vi "状态告警区.vi"(11 "数组":u16[](array[numeric]) format="%04xH") -> (2 "状态告警区 2":T1 {"工作状态" items=["空闲"=0, "水样测试"=1, "标样核查"=2, "零点核查"=3, "跨度核查"=4, "空白测试"=5, "平行样测试"=6, "加标回收"=7, "空白校准"=8, "标样校准"=9, "初始化（清洗）"=10, "单步调试"=254, "简易步骤"=255]; "告警代码" items=["无告警", "缺试剂告警", "缺水样告警", "缺蒸馏水告警", "缺标液告警", "仪表漏液告警", "标定异常告警", "超量程告警", "加热异常", "低试剂预警", "超上限告警", "超下限告警", "仪表内部其他异常", "滴定异常告警", "电极异常告警", "量程切换告警", "参数设置告警", "PH电极电位异常", "电导率电极异常", "浊度光度异常", "溶解氧电极异常", "溶解氧光强异常", "温度异常告警", "PH异常告警", "溶解氧异常告警", "电导率异常告警", "浊度异常告警", "叶绿素异常告警", "藻密度异常告警", "蓝绿藻异常告警", "ORP异常告警", "氨氮异常告警", "清洁刷异常告警", "SD卡异常告警", "蓝牙异常告警", "Wifi异常告警", "流程异常告警"]; "故障代码" items=["无故障", "电机故障", "温度故障", "通讯故障", "滴定故障"]}, 3 "状态告警区":T2 {"工作状态" items=["空闲"=0, "水样测试"=1, "标样核查"=2, "零点核查"=3, "跨度核查"=4, "空白测试"=5, "平行样测试"=6, "加标回收"=7, "空白校准"=8, "标样校准"=9, "初始化（清洗）"=10, "单步调试"=254, "简易步骤"=255]; "告警代码" items=["无告警", "缺试剂告警", "缺水样告警", "缺蒸馏水告警", "缺标液告警", "仪表漏液告警", "标定异常告警", "超量程告警", "加热异常", "低试剂预警", "超上限告警", "超下限告警", "仪表内部其他异常", "滴定异常告警", "电极异常告警", "量程切换告警", "参数设置告警", "PH电极电位异常", "电导率电极异常", "浊度光度异常", "溶解氧电极异常", "溶解氧光强异常", "温度异常告警", "PH异常告警", "溶解氧异常告警", "电导率异常告警", "浊度异常告警", "叶绿素异常告警", "藻密度异常告警", "蓝绿藻异常告警", "ORP异常告警", "氨氮异常告警", "清洁刷异常告警", "SD卡异常告警", "蓝牙异常告警", "Wifi异常告警", "流程异常告警"]; "故障代码" items=["无故障", "电机故障", "温度故障", "通讯故障", "滴定故障"]})   [LabVIEW 2022 SP3, in "斯坦道通用流路CODmn.lvlib"]
panel:
  # "共占用29 WORD"
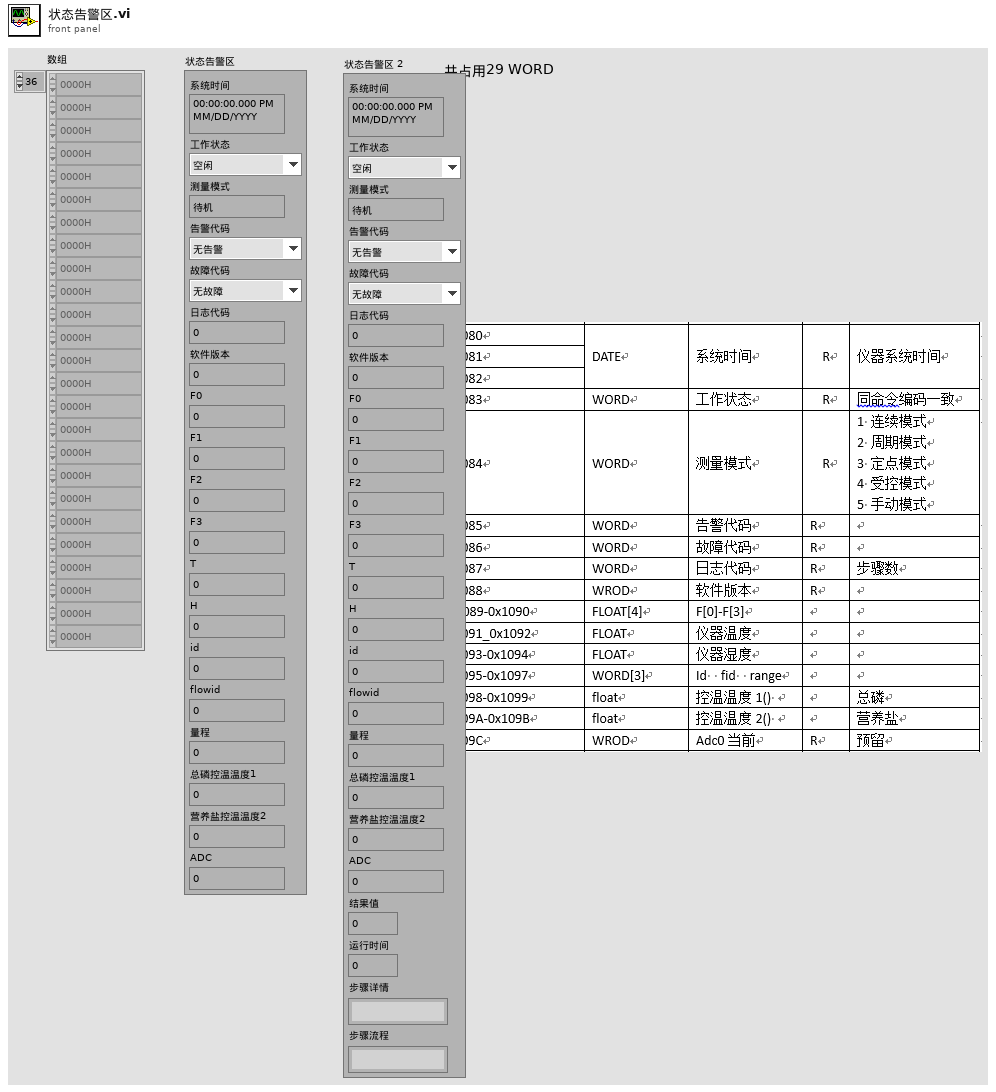
[diagram p1: front panel]
types:
  T1 = cluster{"系统时间":timestamp, "工作状态":u16, "测量模式":enum16{"待机", "连续模式", "周期模式", "定点模式", "受控模式", "手动模式"}, "告警代码":u16, "故障代码":u16, "日志代码":u16, "软件版本":u16, "F0":sgl, "F1":sgl, "F2":sgl, "F3":sgl, "T":sgl, "H":sgl, "id":u16, "flowid":u16, "量程":u16, "总磷控温温度1":sgl, "营养盐控温温度2":sgl, "ADC":sgl, "结果值":sgl, "运行时间":u16, "步骤详情":string, "步骤流程":string}
  T2 = cluster{"系统时间":timestamp, "工作状态":u16, "测量模式":enum16{"待机", "连续模式", "周期模式", "定点模式", "受控模式", "手动模式"}, "告警代码":u16, "故障代码":u16, "日志代码":u16, "软件版本":u16, "F0":sgl, "F1":sgl, "F2":sgl, "F3":sgl, "T":sgl, "H":sgl, "id":u16, "flowid":u16, "量程":u16, "总磷控温温度1":sgl, "营养盐控温温度2":sgl, "ADC":sgl}
  T3 = enum16{"待机", "连续模式", "周期模式", "定点模式", "受控模式", "手动模式"}
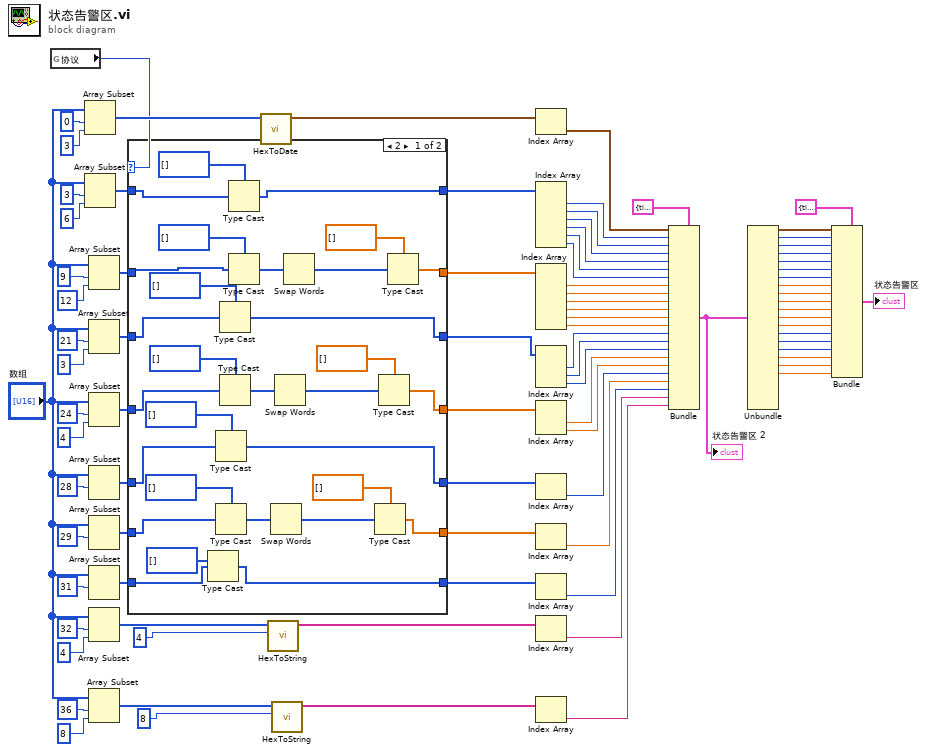
[diagram p0: block diagram]
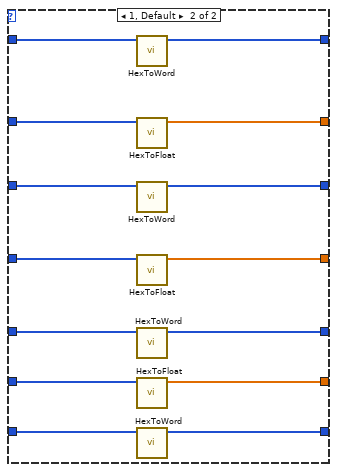
[diagram p2: hidden frame]
diagram:
  n1 = global read "总磷总氮断电保存全局变量.vi" "协议"() -> (w1:u16)
  n2 = Array Subset(array="数组", index=0 ("索引"), length=3 ("长度")) -> (w85:u16[])
  n3 = Array Subset(array="数组", index=3 ("索引"), length=6 ("长度")) -> (w80:u16[])
  n4 = Array Subset(array="数组", index=9 ("索引"), length=12 ("长度")) -> (w70:u16[])
  n5 = Array Subset(array="数组", index=21 ("索引"), length=3 ("索引")) -> (w60:u16[])
  n6 = Array Subset(array="数组", index=24 ("索引"), length=4 ("索引")) -> (w53:u16[])
  n7 = Array Subset(array="数组", index=28 ("索引")) -> (w48:u16[])  [unwired: 1 in]
  n8 = Array Subset(array="数组", index=29 ("索引")) -> (w21:u16[])  [unwired: 1 in]
  n9 = Array Subset(array="数组", index=31 ("索引")) -> (w17:u16[])  [unwired: 1 in]
  n10 = Array Subset(array="数组", index=32 ("索引"), length=4 ("长度")) -> (w13:u16[])
  n11 = Array Subset(array="数组", index=36 ("索引"), length=8 ("长度")) -> (w5:u16[])
  n12 = case shown="2" w1 {
    tunnel: w80 -> [w101 w131]
    tunnel: [w100 w130] -> w79
    tunnel: w70 -> [w98 w129]
    tunnel: [w99 w128] -> w69
    tunnel: w60 -> [w97 w127]
    tunnel: [w96 w126] -> w59
    tunnel: w53 -> [w95 w125]
    tunnel: [w94 w124] -> w52
    tunnel: [w92 w123] -> w49
    tunnel: w48 -> [w93 w122]
    tunnel: w21 -> [w91 w121]
    tunnel: [w90 w120] -> w20
    tunnel: w17 -> [w89 w119]
    tunnel: [w88 w118] -> w16
    frame 2 {
      n13 = Type Cast(type=u16[] [], x=w89) -> (*(type *) &x=w88:u16[])
      n14 = Type Cast(type=u16[] [], x=w93) -> (*(type *) &x=w92:u16[])
      n15 = Type Cast(type=i32[] [], x=w91) -> (*(type *) &x=w105:i32[])
      n16 = Type Cast(type=u16[] [], x=w97) -> (*(type *) &x=w96:u16[])
      n17 = Type Cast(type=i32[] [], x=w95) -> (*(type *) &x=w110:i32[])
      n18 = Type Cast(type=u16[] [], x=w101) -> (*(type *) &x=w100:u16[])
      n19 = Type Cast(type=i32[] [], x=w98) -> (*(type *) &x=w115:i32[])
      n20 = Swap Words(1:w105) -> (0:w103:i32[])
      n21 = Swap Words(1:w110) -> (0:w108:i32[])
      n22 = Swap Words(1:w115) -> (0:w113:i32[])
      n23 = Type Cast(type=sgl[] [], x=w103) -> (*(type *) &x=w90:sgl[])
      n24 = Type Cast(type=sgl[] [], x=w108) -> (*(type *) &x=w94:sgl[])
      n25 = Type Cast(type=sgl[] [], x=w113) -> (*(type *) &x=w99:sgl[])
    }
    frame 1, Default {
      n26 = call "HexToWord.vi"("数组"=w131) -> ("WORD"=w130:u16[])  [unwired: 10 in]
      n27 = call "HexToFloat.vi"("数组"=w129) -> ("FLOAT"=w128:sgl[])  [unwired: 10 in]
      n28 = call "HexToWord.vi"("数组"=w127) -> ("WORD"=w126:u16[])  [unwired: 10 in]
      n29 = call "HexToFloat.vi"("数组"=w125) -> ("FLOAT"=w124:sgl[])  [unwired: 10 in]
      n30 = call "HexToWord.vi"("数组"=w122) -> ("WORD"=w123:u16[])  [unwired: 10 in]
      n31 = call "HexToFloat.vi"("数组"=w121) -> ("FLOAT"=w120:sgl[])  [unwired: 10 in]
      n32 = call "HexToWord.vi"("数组"=w119) -> ("WORD"=w118:u16[])  [unwired: 10 in]
    }
  }
  n33 = call "HexToDate.vi"("数组"=w85) -> ("DATE"=w82:timestamp[])  [unwired: 10 in]
  n34 = call "HexToString.vi"("字符个数"=4, "数组"=w13) -> ("STRING"=w11:string[])  [unwired: 9 in]
  n35 = call "HexToString.vi"("字符个数"=8, "数组"=w5) -> ("STRING"=w7:string[])  [unwired: 9 in]
  n36 = Index Array(array=w82) -> (element=w81:timestamp)  [unwired: 1 in]
  n37 = Index Array(array=w79) -> (element #1=w78:u16, element #2=w77:u16, element #3=w76:u16, element #4=w75:u16, element #5=w74:u16, element #6=w73:u16)  [unwired: 6 in]
  n38 = Index Array(array=w69) -> (element #1=w68:sgl, element #2=w67:sgl, element #3=w66:sgl, element #4=w65:sgl, element #5=w64:sgl, element #6=w63:sgl)  [unwired: 6 in]
  n39 = Index Array(array=w59) -> (element #1=w58:u16, element #2=w57:u16, element #3=w56:u16)  [unwired: 3 in]
  n40 = Index Array(array=w52) -> (element #1=w51:sgl, element #2=w50:sgl)  [unwired: 2 in]
  n41 = Index Array(array=w49) -> (element=w46:u16)  [unwired: 1 in]
  n42 = Index Array(array=w20) -> (element=w19:sgl)  [unwired: 1 in]
  n43 = Index Array(array=w16) -> (element=w15:u16)  [unwired: 1 in]
  n44 = Index Array(array=w11) -> (element=w10:string)  [unwired: 1 in]
  n45 = Index Array(array=w7) -> (element=w2:string)  [unwired: 1 in]
  n46 = Bundle(cluster=T1 {"系统时间"=timestamp(0 s since 1904-01-01), "工作状态"=0, "测量模式"=enum."待机", "告警代码"=0, "故障代码"=0, "日志代码"=0, "软件版本"=0, "F0"=0.0, "F1"=0.0, "F2"=0.0, "F3"=0.0, "T"=0.0, "H"=0.0, "id"=0, "flowid"=0, "量程"=0, "总磷控温温度1"=0.0, "营养盐控温温度2"=0.0, "ADC"=0.0, "结果值"=0.0, "运行时间"=0, "步骤详情"="", "步骤流程"=""} ("状态告警区 2"), "系统时间"=w81, "工作状态"=w78, "测量模式"=w77, "告警代码"=w76, "故障代码"=w75, "日志代码"=w74, "软件版本"=w73, "F0"=w68, "F1"=w67, "F2"=w66, "F3"=w65, "T"=w64, "H"=w63, "id"=w58, "flowid"=w57, "量程"=w56, "总磷控温温度1"=w51, "营养盐控温温度2"=w50, "ADC"=w46, "结果值"=w19, "运行时间"=w15, "步骤详情"=w10, "步骤流程"=w2) -> (w44:T1)
  "状态告警区 2" <- w44
  n47 = Unbundle(w44) -> ("系统时间"=w42:timestamp, "工作状态"=w41:u16, "测量模式"=w40:T3, "告警代码"=w39:u16, "故障代码"=w38:u16, "日志代码"=w37:u16, "软件版本"=w36:u16, "F0"=w35:sgl, "F1"=w34:sgl, "F2"=w33:sgl, "F3"=w32:sgl, "T"=w31:sgl, "H"=w30:sgl, "id"=w29:u16, "flowid"=w28:u16, "量程"=w27:u16, "总磷控温温度1"=w26:sgl, "营养盐控温温度2"=w25:sgl, "ADC"=w24:sgl)  [unwired: 4 out]
  n48 = Bundle(cluster=T2 {"系统时间"=timestamp(0 s since 1904-01-01), "工作状态"=0, "测量模式"=enum."待机", "告警代码"=0, "故障代码"=0, "日志代码"=0, "软件版本"=0, "F0"=0.0, "F1"=0.0, "F2"=0.0, "F3"=0.0, "T"=0.0, "H"=0.0, "id"=0, "flowid"=0, "量程"=0, "总磷控温温度1"=0.0, "营养盐控温温度2"=0.0, "ADC"=0.0} ("状态告警区"), "系统时间"=w42, "工作状态"=w41, "测量模式"=w40, "告警代码"=w39, "故障代码"=w38, "日志代码"=w37, "软件版本"=w36, "F0"=w35, "F1"=w34, "F2"=w33, "F3"=w32, "T"=w31, "H"=w30, "id"=w29, "flowid"=w28, "量程"=w27, "总磷控温温度1"=w26, "营养盐控温温度2"=w25, "ADC"=w24) -> (→"状态告警区":T2)
